vi "VIs to Ignore.vi"() -> (3 "VIs to Ignore":string[](array[string]))   [LabVIEW 2020, in "Peek Window.lvlib"]
uses:
  Peek Window.lvlib
  Main.vi
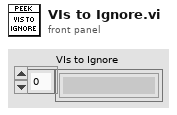
[diagram p1: front panel]
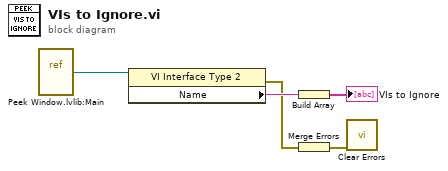
[diagram p0: block diagram]
diagram:
  n1 = vi-ref "Peek Window.lvlib:Main.vi"() -> (w5:refnum<vi>)
  n2 = property class="VI Interface Type 2"(reference=w5) -> (error out=w2:errorcluster, "Name"=w4:string)  [unwired: 1 in, 1 out]
  n3 = Build Array(w4) -> (→"VIs to Ignore":string[])
  n4 = Merge Errors(w2) -> (w1:errorcluster)
  n5 = call <vilib>:"Clear Errors.vi"("error in (no error)"=w1) -> ()  [unwired: 5 in, 2 out]
